vi "Inspect Fiducials.vi"(7 "Console Log in":refnum<class "Console Log.lvclass">, 8 "error in":errorcluster, 11 "Gluing Procedure in":refnum<class "Gluing Procedure.lvclass">) -> (0 "error out":errorcluster, 1 "Step canceled?":bool, 3 "Gluing Procedure out":refnum<class "Gluing Procedure.lvclass">, 5 "Console Log out":refnum<class "Console Log.lvclass">)   [LabVIEW 2011, in "Gluing Procedure.lvclass"]
uses:
  Gluing Procedure.lvclass
  Application Utilities/Console Log/Console Log.lvclass
  Type Definitions/Inspect Fuducials.ctl
  Shared Components/Utils/Type Definitions/Part Fiducials.ctl
  Shared Components/Utils/Type Definitions/Fiducial Image.ctl
  Shared Components/Utils/Type Definitions/Physical Image.ctl
  Shared Components/Vec3d Class/Vec3d Class.lvclass
  <vilib>/vision/Image Controls.llb/IMAQ Image.ctl
  Shared Components/Utils/Type Definitions/Fiducial with Source.ctl
  Shared Components/Gantry Class/Gantry Class.lvclass
  Shared Components/CameraTool Class/CameraTool Class.lvclass
panel:
  # "This VI needs to load the camera and inspect fiducials\nfor selected chuck/slots for HDIs, Stamps, Weights, and BBMs\n\nTo think about:\nShould split up HDI, Stamp, Weight, and BBMs into their own sub VIs, where this one calls them?"
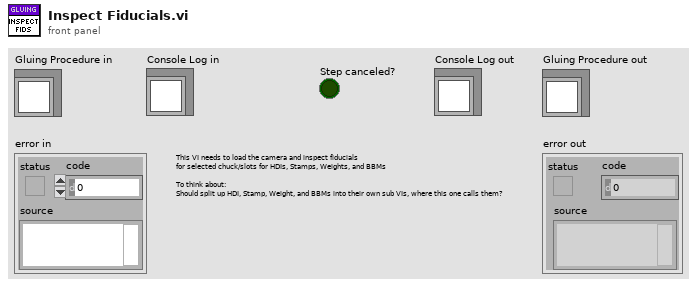
[diagram p1: front panel]
types:
  T1 = typedef "Inspect Fuducials.ctl" = cluster{"Path Fiducials":cluster{"HDI Fiducials":T2, "Stamp Fiducials":T2, "Weight Fiducials":T2, "BBM Fiducials":T2}[], "Has been run?":bool}
  T2 = typedef "Part Fiducials.ctl" = cluster{"Fiducials":T3[], "Chuck":i32, "Slot":i32}
  T3 = typedef "Fiducial Image.ctl" = cluster{"Fiducial Image":T4, "Selected Fiducial":T6, "fiducial name":string}
  T4 = typedef "Physical Image.ctl" = cluster{"Image Position":refnum<class "Vec3d Class.lvclass">, "Image Reference":T5, "Field of View":cluster{"x(mm)":dbl, "y(mm)":dbl}}
  T5 = typedef "IMAQ Image.ctl" = refnum<image>
  T6 = typedef "Fiducial with Source.ctl" = cluster{"Fiducial Image Coordinate":refnum<class "Vec3d Class.lvclass">, "Fiducial Source":enum16{"Pattern Recognition", "User", "Error", "Default"}}
  T7 = cluster{"HDI Fiducials":T2, "Stamp Fiducials":T2, "Weight Fiducials":T2, "BBM Fiducials":T2}
  T8 = typedef "Configure.ctl" = cluster{"Has been run?":bool, "Active Paths":T9, "Glue Pathways":T10, "Chuck Module Used for BBM:":T12}
  T9 = typedef "Active Paths.ctl" = bool[]
  T10 = typedef "Glue Paths.ctl" = T11[]
  T11 = typedef "Glue Path.ctl" = cluster{"HDI Slot ":i32, "Stamp Slot":i32, "Glue Slot":i32, "Weight Slot":i32, "BBM Slot":i32}
  T12 = typedef "BBM Chuck Used.ctl" = i32
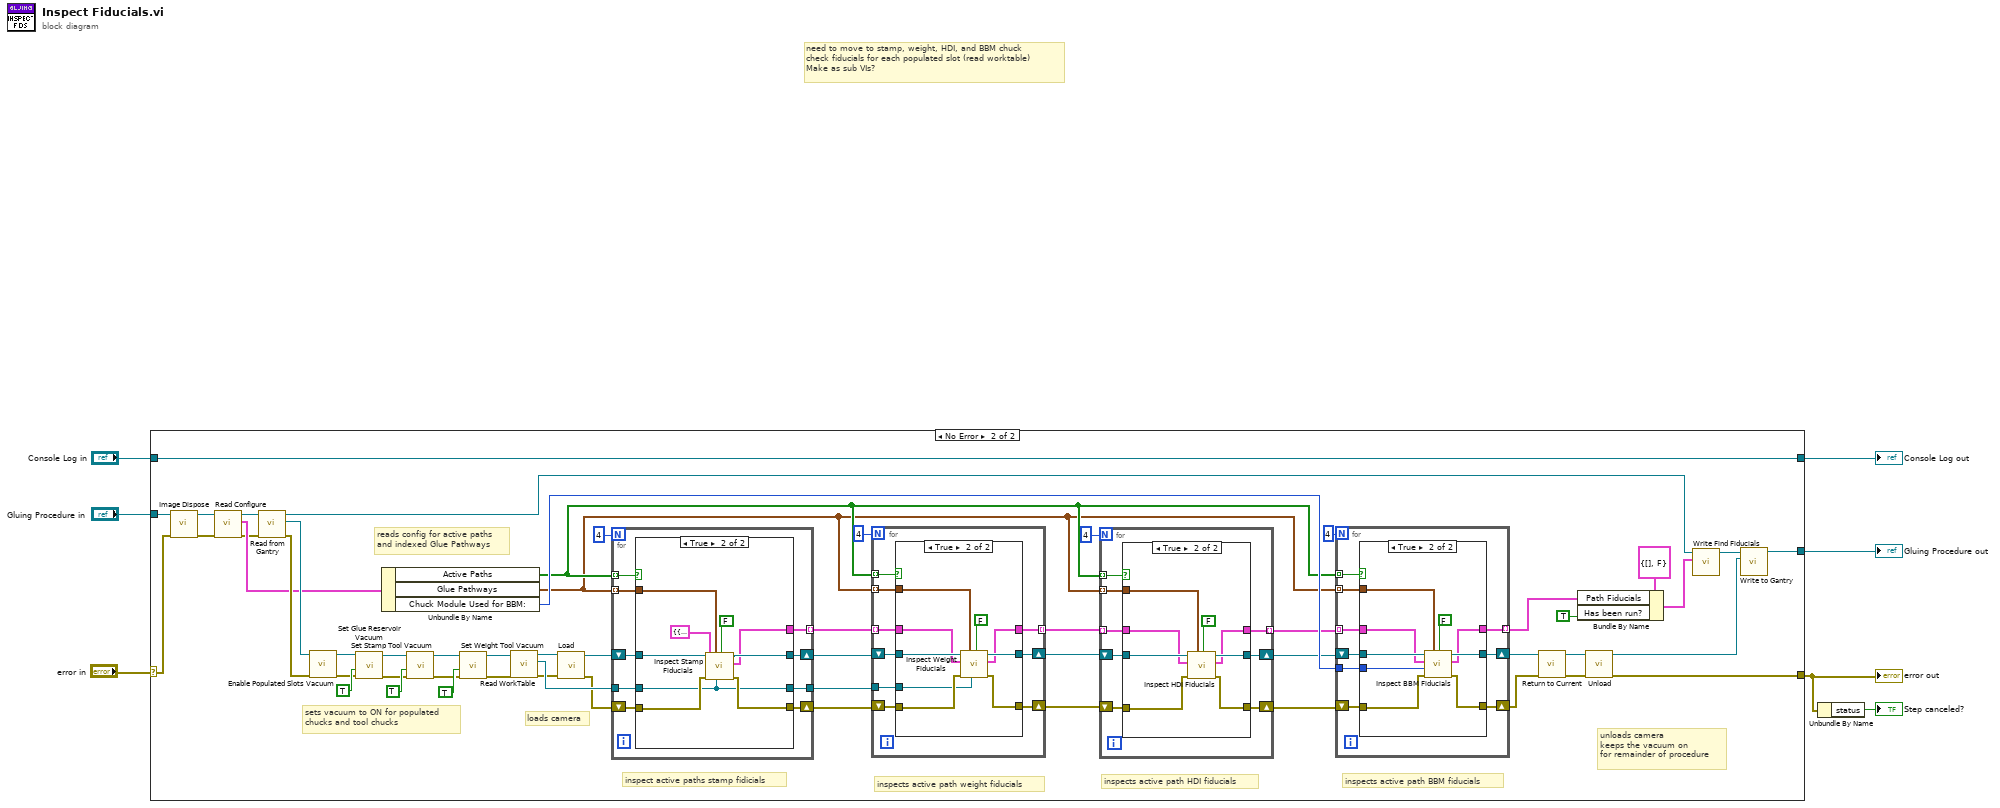
[diagram p0: block diagram]
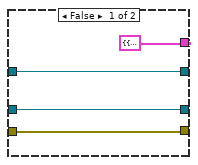
[diagram p6: hidden frame]
diagram:
  # "need to move to stamp, weight, HDI, and BBM chuck\ncheck fiducials for each populated slot (read worktable)\nMake as sub VIs?"
  n1 = case shown="No Error" "error in" {
    selector: "error in" -> [w9 w65]
    tunnel: "Gluing Procedure in" -> [w10 w66]
    tunnel: [w10 w28] -> w5
    tunnel: [w9 w15] -> w3
    tunnel: [w8 w17] -> w4
    tunnel: "Console Log in" -> [w8 w17]
    frame Error {
    }
    frame No Error {
      # "loads camera"
      # "unloads camera\nkeeps the vacuum on\nfor remainder of procedure"
      # "inspects active path BBM fiducials"
      # "inspects active path HDI fiducials"
      # "reads config for active paths\nand indexed Glue Pathways"
      # "inspects active path weight fiducials"
      # "inspect active paths stamp fidicials"
      # "sets vacuum to ON for populated\nchucks and tool chucks"
      n2 = call "Image Dispose.vi"("error in"=w65, "Gluing Procedure in"=w66) -> ("error out"=w27:errorcluster, "Gluing Procedure out"=w52:refnum<class "Gluing Procedure.lvclass">)  [unwired: 8 in]
      n3 = call "Read Configure.vi"("error in (no error)"=w27, "Gluing Procedure in"=w52) -> ("error out"=w26:errorcluster, "Configure"=w50:T8, "Gluing Procedure out"=w51:refnum<class "Gluing Procedure.lvclass">)  [unwired: 7 in]
      n4 = call "Read from Gantry.vi"("error in (no error)"=w26, "Gluing Procedure in"=w51) -> ("error out"=w63:errorcluster, "Gantry"=w64:refnum<class "Gantry Class.lvclass">, "Gluing Procedure out"=w19:refnum<class "Gluing Procedure.lvclass">)  [unwired: 7 in]
      n5 = call-dynamic "Enable Populated Slots Vacuum.vi"("error in"=w63, "Gantry in"=w64) -> ("error out"=w25:errorcluster, "Gantry out"=w60:refnum<class "Gantry Class.lvclass">)  [unwired: 8 in]
      n6 = call-dynamic "Set Glue Reservoir Vacuum.vi"("error in (no error)"=w25, "On/Off"=TRUE, "Gantry Class in"=w60) -> ("error out"=w24:errorcluster, "Gantry Class out"=w58:refnum<class "Gantry Class.lvclass">)  [unwired: 7 in]
      n7 = Unbundle By Name(w50) -> ("Active Paths"=w38:T9, "Glue Pathways"=w37:T10, "Chuck Module Used for BBM:"=w42:T12)
      n8 = call-dynamic "Set Stamp Tool Vacuum.vi"("error in"=w24, "On/Off"=TRUE, "Gantry in"=w58) -> ("error out"=w23:errorcluster, "Gantry out"=w56:refnum<class "Gantry Class.lvclass">)  [unwired: 7 in]
      n9 = call-dynamic "Set Weight Tool Vacuum.vi"("error in"=w23, "On/Off"=TRUE, "Gantry in"=w56) -> ("error out"=w22:errorcluster, "Gantry out"=w54:refnum<class "Gantry Class.lvclass">)  [unwired: 7 in]
      n10 = call-dynamic "Read WorkTable.vi"("error in"=w22, "Gantry Class in"=w54) -> ("error out"=w21:errorcluster, "WorkTable Class.lvclass"=w53:refnum<class "WorkTable Class.lvclass">, "Gantry Class out"=w62:refnum<class "Gantry Class.lvclass">)  [unwired: 7 in]
      n11 = call "Load.vi"("error in"=w21, "Gantry In"=w62) -> ("error out"=w47:errorcluster, "CameraTool out"=w61:refnum<class "CameraTool Class.lvclass">)  [unwired: 8 in]
      n12 = for {
        N: 4 -> [_]
        tunnel: w53 -> [w135]
        tunnel: w38 -> [w134] mode=indexing
        shift-right: [w131] -> w45
        shift-left: w61 -> [w136]
        tunnel: w37 -> [w133] mode=indexing
        tunnel: [w132] -> w46 mode=indexing
        shift-right: [w129] -> w44
        shift-left: w47 -> [w130]
        tunnel: [w128] -> w43
        n13 = case shown="True" w134 {
          tunnel: w136 -> [w140 w149]
          tunnel: w135 -> [w139 w144]
          tunnel: w133 -> [_ w148]
          tunnel: [T7 {"HDI Fiducials"={"Fiducials"=[], "Chuck"=0, "Slot"=0}, "Stamp Fiducials"={"Fiducials"=[], "Chuck"=0, "Slot"=0}, "Weight Fiducials"={"Fiducials"=[], "Chuck"=0, "Slot"=0}, "BBM Fiducials"={"Fiducials"=[], "Chuck"=0, "Slot"=0}} ("Single Path in") w142] -> w132
          tunnel: [w140 w143] -> w131
          tunnel: w130 -> [w138 w146]
          tunnel: [w138 w145] -> w129
          tunnel: [w139 w144] -> w128
          frame False {
          }
          frame True {
            n14 = call "Inspect Stamp Fiducials.vi"("Dispose Images?"=FALSE, "WorkTable Class in"=w144, "Glue Pathways"=w148, "error in"=w146, "Single Path in"=T7 {"HDI Fiducials"={"Fiducials"=[], "Chuck"=0, "Slot"=0}, "Stamp Fiducials"={"Fiducials"=[], "Chuck"=0, "Slot"=0}, "Weight Fiducials"={"Fiducials"=[], "Chuck"=0, "Slot"=0}, "BBM Fiducials"={"Fiducials"=[], "Chuck"=0, "Slot"=0}}, "CameraTool in"=w149) -> ("error out"=w145:errorcluster, "Single Path out"=w142:T7, "CameraTool out"=w143:refnum<class "CameraTool Class.lvclass">)  [unwired: 3 in]
          }
        }
      }
      n15 = for {
        N: 4 -> [_]
        tunnel: w43 -> [w114]
        tunnel: w38 -> [w113] mode=indexing
        shift-right: [w109] -> w40
        shift-left: w45 -> [w115]
        tunnel: w46 -> [w112] mode=indexing
        tunnel: w37 -> [w111] mode=indexing
        tunnel: [w110] -> w41 mode=indexing
        shift-right: [w107] -> w39
        shift-left: w44 -> [w108]
        n16 = case shown="True" w113 {
          tunnel: w115 -> [w117 w122]
          tunnel: w114 -> [_ w119]
          tunnel: w112 -> [w118 w121]
          tunnel: w111 -> [_ w127]
          tunnel: [w118 w120] -> w110
          tunnel: [w117 w125] -> w109
          tunnel: w108 -> [w116 w123]
          tunnel: [w116 w124] -> w107
          frame False {
          }
          frame True {
            n17 = call "Inspect Weight Fiducials.vi"("Dispose Images?"=FALSE, "WorkTable Class in"=w119, "Glue Pathways"=w127, "error in"=w123, "Single Path in"=w121, "CameraTool in"=w122) -> ("error out"=w124:errorcluster, "Single Path out"=w120:T7, "CameraTool out"=w125:refnum<class "CameraTool Class.lvclass">)  [unwired: 3 in]
          }
        }
      }
      n18 = for {
        N: 4 -> [_]
        tunnel: w38 -> [w73] mode=indexing
        shift-right: [w69] -> w35
        shift-left: w40 -> [w74]
        tunnel: w41 -> [w72] mode=indexing
        tunnel: w37 -> [w71] mode=indexing
        tunnel: [w70] -> w36 mode=indexing
        shift-right: [w67] -> w34
        shift-left: w39 -> [w68]
        n19 = case shown="True" w73 {
          tunnel: w74 -> [w76 w80]
          tunnel: w72 -> [w77 w79]
          tunnel: w71 -> [_ w85]
          tunnel: [w77 w78] -> w70
          tunnel: [w76 w83] -> w69
          tunnel: w68 -> [w75 w81]
          tunnel: [w75 w82] -> w67
          frame False {
          }
          frame True {
            n20 = call "Inspect HDI Fiducials.vi"("Dispose Images?"=FALSE, "Glue Pathways"=w85, "error in"=w81, "Single Path in"=w79, "CameraTool in"=w80) -> ("error out"=w82:errorcluster, "Single Path out"=w78:T7, "CameraTool out"=w83:refnum<class "CameraTool Class.lvclass">)  [unwired: 4 in]
          }
        }
      }
      n21 = for {
        N: 4 -> [_]
        tunnel: w38 -> [w93] mode=indexing
        shift-right: [w89] -> w32
        shift-left: w35 -> [w94]
        tunnel: w36 -> [w92] mode=indexing
        tunnel: w37 -> [w91] mode=indexing
        tunnel: [w90] -> w33 mode=indexing
        shift-right: [w87] -> w30
        shift-left: w34 -> [w88]
        tunnel: w42 -> [w86]
        n22 = case shown="True" w93 {
          tunnel: w94 -> [w96 w101]
          tunnel: w92 -> [w97 w98]
          tunnel: w91 -> [_ w106]
          tunnel: [w97 w100] -> w90
          tunnel: [w96 w104] -> w89
          tunnel: w88 -> [w95 w102]
          tunnel: [w95 w103] -> w87
          tunnel: w86 -> [_ w99]
          frame False {
          }
          frame True {
            n23 = call "Inspect BBM Fiducials.vi"("Dispose Images?"=FALSE, "Glue Pathways"=w106, "error in"=w102, "BBM Chuck"=w99, "Single Path in"=w98, "CameraTool in"=w101) -> ("error out"=w103:errorcluster, "Single Path out"=w100:T7, "CameraTool out"=w104:refnum<class "CameraTool Class.lvclass">)  [unwired: 3 in]
          }
        }
      }
      n24 = call-dynamic "Return to Current.vi"("error in"=w30, "Gantry in"=w32) -> ("error out"=w29:errorcluster, "Gantry out"=w31:refnum<class "CameraTool Class.lvclass">)  [unwired: 8 in]
      n25 = Bundle By Name(cluster=T1 {"Path Fiducials"=[], "Has been run?"=FALSE} ("Find Fiducials"), "Path Fiducials"=w33, "Has been run?"=TRUE) -> (w20:T1)
      n26 = call "Unload.vi"("error in"=w29, "CameraTool in"=w31) -> ("error out"=w15:errorcluster, "Gantry out"=w16:refnum<class "Gantry Class.lvclass">)  [unwired: 8 in]
      n27 = call "Write Find Fiducials.vi"("Find Fiducials"=w20, "Gluing Procedure in"=w19) -> ("Gluing Procedure out"=w18:refnum<class "Gluing Procedure.lvclass">)  [unwired: 8 in, 1 out]
      n28 = call "Write to Gantry.vi"("Gantry"=w16, "Gluing Procedure in"=w18) -> ("Gluing Procedure out"=w28:refnum<class "Gluing Procedure.lvclass">)  [unwired: 8 in, 1 out]
    }
  }
  "error out" <- w3
  "Gluing Procedure out" <- w5
  "Console Log out" <- w4
  n29 = Unbundle By Name(w3) -> ("status"=→"Step canceled?":bool)
